vi "Future Usage - Cancel Long Operation.vi"   [LabVIEW 2017]
uses:
  Futures/Futures.lvlib
  Futures/Future/Future.lvclass
  Futures/Promise/Promise.lvclass
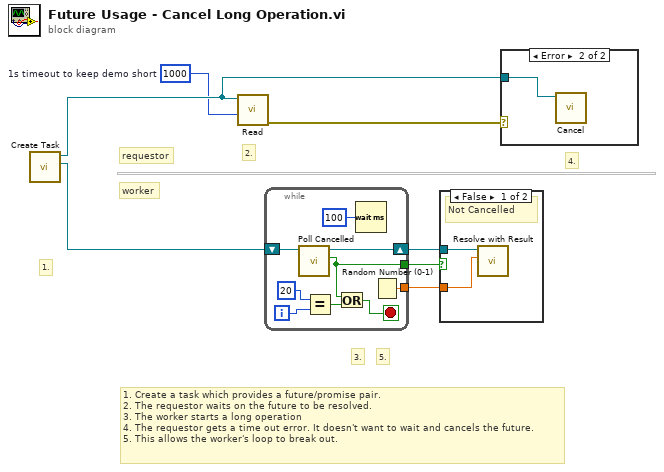
[diagram p0: block diagram]
diagram:
  w5 = 1000  # 1s timeout to keep demo short
  # "5."
  # "3."
  # "4."
  # "2."
  # "1. Create a task which provides a future/promise pair.\n2. The requestor waits on the future to be resolved.\n3. The worker starts a long operation\n4. The requestor gets a time out error. It doesn't want to wait and cancels the future.\n5. This allows the worker's loop to break out."
  # "requestor"
  # "worker"
  # "1."
  n1 = call "Create Task.vi"() -> ("Promise out"=w3:refnum<class "Promise.lvclass">, "Future out"=w6:refnum<class "Future.lvclass">)  [unwired: 9 in, 1 out]
  n2 = call "Read.vi"("timeout in ms (60 sec)"=w5, "Future in"=w6) -> ("error out"=w7:errorcluster)  [unwired: 6 in, 3 out]
  n3 = while {
    tunnel: [w16] -> w4
    shift-right: [w14] -> w2
    shift-left: w3 -> [w15]
    tunnel: [w10] -> w1
    i -> [w12]
    stop <- w8 stop-if-true
    n4 = call "Poll Cancelled.vi"("Promise in"=w15) -> ("Cancelled"=w10:bool, "Promise out"=w14:refnum<class "Promise.lvclass">)  [unwired: 8 in, 1 out]
    n5 = Equal?(x=20, y=w12) -> (x = y?=w9:bool)
    n6 = Or(x=w10, y=w9) -> (x .or. y?=w8:bool)
    n7 = Wait (ms)(milliseconds to wait=u32 100) -> ()  [unwired: 1 out]
    n8 = Random Number (0-1)() -> (number: 0 to 1=w16:dbl)
  }
  n9 = case shown="False" w1 {
    tunnel: w4 -> [w18 _]
    tunnel: w2 -> [w17 _]
    frame False {
      # "Not Cancelled"
      n10 = call "Resolve with Result.vi"("Result"=w18, "Promise in"=w17) -> ()  [unwired: 9 in, 1 out]
    }
    frame True {
      # "Cancelled -\nDo Nothing"
    }
  }
  n11 = case shown="Error" w7 {
    tunnel: w6 -> [_ w19]
    frame No Error {
    }
    frame Error {
      n12 = call "Cancel.vi"("Future in"=w19) -> ()  [unwired: 10 in, 1 out]
    }
  }
